vi "Offset_Loop.vi"(0 "Port":u16, 1 "LV_Variables":T1={"ACQPS"=25, "Config_Enable"=1, "Prescale"=1, "ADC"=enum."A", "Adc_Channel"=1, "Ref_Int/EXT"=FALSE}, 2 "ACQPS":u16[](array[numeric]), 5 "Core":u16, 7 "Pin_Config":i32, 11 "error in":errorcluster, 12 "Voltage":dbl[](array[numeric]), 14 "VREF_Measured":dbl=2.5 format="%#_13g") -> (4 "Port Number out":u16, 6 "Core Number out":u16, 8 "output array":string[][](array[string]), 13 "OFF+GAIN":string[][](array[string]), 15 "error out":errorcluster)   [LabVIEW 2019]
uses:
  Ctrls/ADC_LV_Variables.ctl
  Ctrls/ADC_CTRL.ctl
  <userlib>/_TI-LA/Reusable/CCS/APIs/Data/Polymorphics/Write Data To Symbol - U16.vi
  <userlib>/_TI-LA/Reusable/CCS/APIs/CCS.lvlib
  <vilib>/Analysis/NI_AALBase.lvlib
  common/Comman_nilesh/File_Write/Data_Logging.lvclass
  <userlib>/_TI-LA/Instr Drivers/Multimeter/Agilent 3446X Series/Agilent 3446X Series.lvlib
panel:
  out "AVG":dbl format="%0.2f"
  out "Array":dbl[](array[numeric])
  out "LV_Variables_out":T1={"ACQPS"=25, "Config_Enable"=1, "Prescale"=1, "ADC"=enum."A", "Adc_Channel"=1, "Ref_Int/EXT"=FALSE}
  in  "VISA_SGEN":refnum<visa-resource-name>="USB0::0x0957::0x1607::MY50001293::INSTR"
  out "standard deviation":dbl format="%0.2f"
  out "mean":dbl format="%0.2f"
  out "Waveform Graph":u16[](graph)
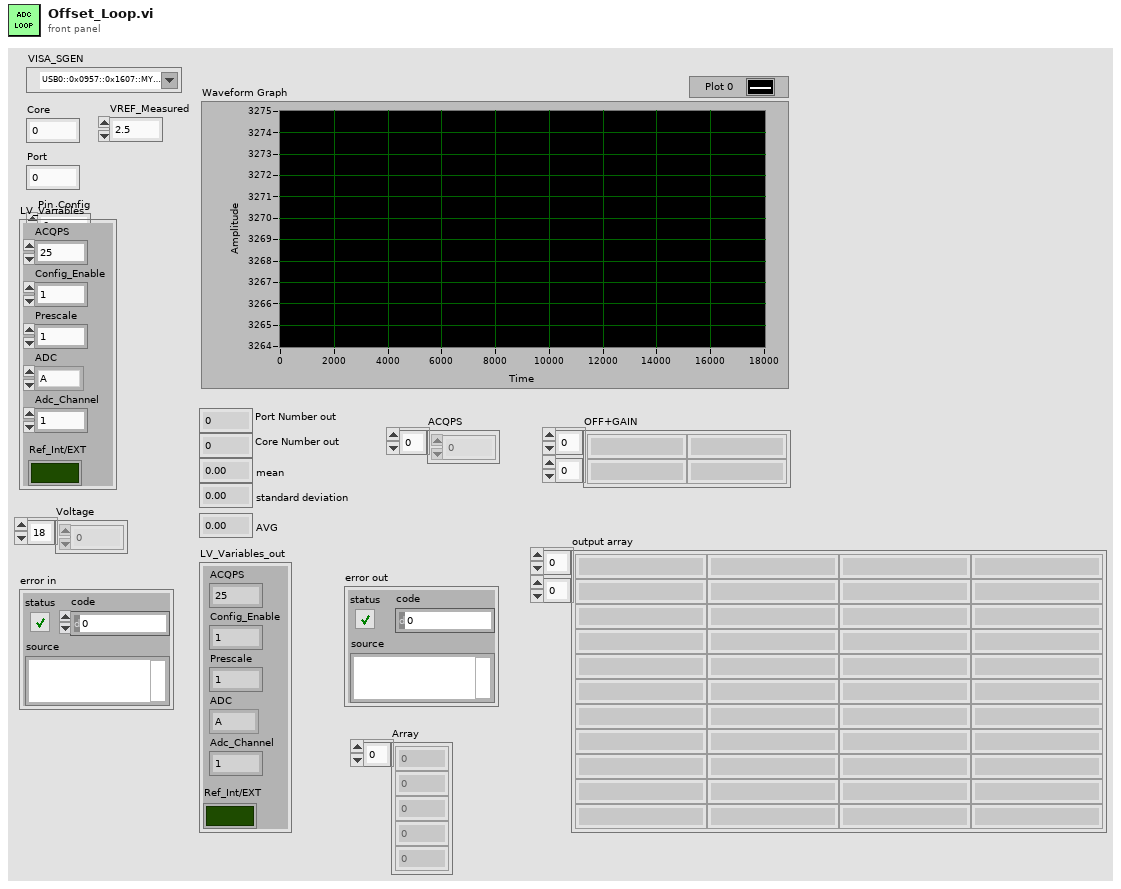
[diagram p1: front panel]
types:
  T1 = typedef "ADC_LV_Variables.ctl" = cluster{"ACQPS":u16, "Config_Enable":u16, "Prescale":u16, "ADC":T2, "Adc_Channel":u16, "Ref_Int/EXT":bool}
  T2 = typedef "ADC_CTRL.ctl" = enum16{"A", "B", "C"}
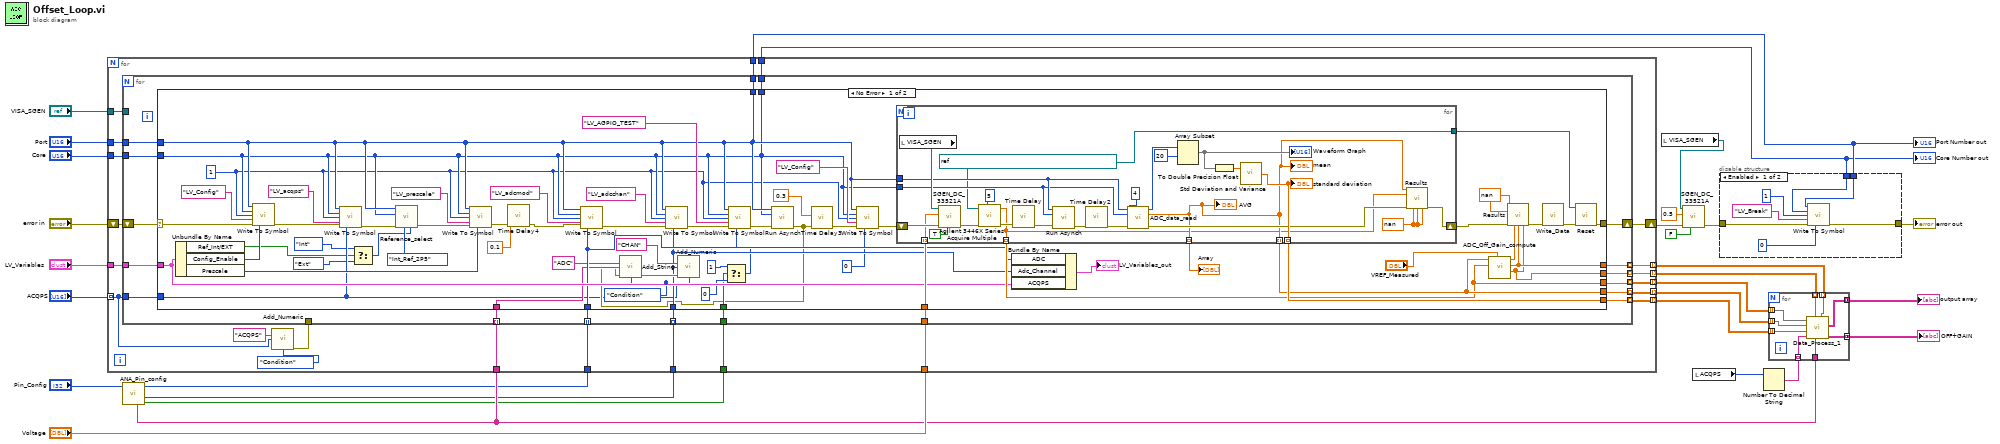
[diagram p0: block diagram]
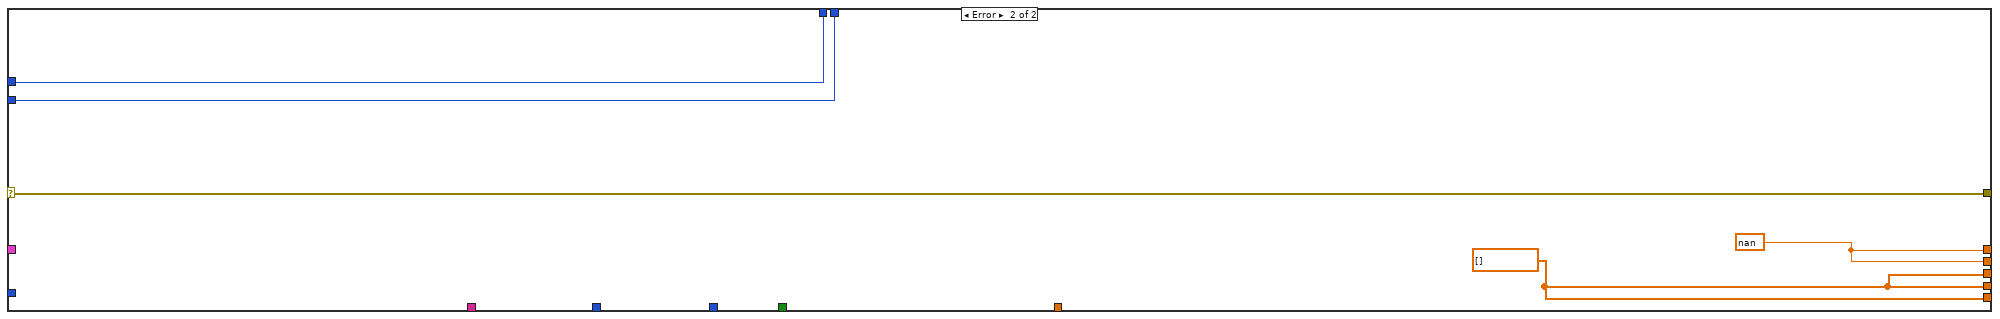
[diagram p3: hidden frame]
diagram:
  n1 = call "ANA_Pin_config.vi"("Pin_Config"="Pin_Config") -> ("Boolean"=w8:bool, "ADC_Channel"=w1:u16[], "ADC"=w2:T2[], "ADC+CH"=w9:string[])  [unwired: 7 in]
  n2 = for {
    tunnel: "Port" -> [w51]
    tunnel: "Core" -> [w50]
    tunnel: "LV_Variables" -> [w49]
    tunnel: [w47] -> w24
    tunnel: [w46] -> w23
    tunnel: w2 -> [w45]
    tunnel: w1 -> [w44]
    tunnel: "VISA_SGEN" -> [w43]
    tunnel: [w42] -> w10 mode=indexing
    tunnel: "Voltage" -> [w41]
    tunnel: [w40] -> w11 mode=indexing
    tunnel: [w39] -> w19 mode=indexing
    tunnel: [w38] -> w18 mode=indexing
    tunnel: [w37] -> w17 mode=indexing
    shift-right: [w48] -> w7
    shift-left: "error in" -> [w32]
    tunnel: "ACQPS" -> [w34] mode=indexing
    tunnel: w9 -> [w33]
    tunnel: w8 -> [w30]
    n3 = call "Add_Numeric.vi"("Name"="ACQPS", "Numeric_FC"=w34, "Type"=enum16{"Result", "Condition"}."Condition") -> ("error out"=w31:errorcluster)  [unwired: 11 in, 1 out]
    n4 = for {
      tunnel: w51 -> [w66]
      tunnel: w50 -> [w67]
      tunnel: w49 -> [w68]
      shift-right: [w69] -> w48
      shift-left: w32 -> [w63]
      tunnel: [w64] -> w46
      tunnel: [w65] -> w47
      tunnel: w45 -> [w55] mode=indexing
      tunnel: w44 -> [w62] mode=indexing
      tunnel: [w61] -> w38 mode=indexing
      tunnel: [w60] -> w37 mode=indexing
      tunnel: w41 -> [w59]
      tunnel: w43 -> [_]
      tunnel: [w58] -> w42 mode=indexing
      tunnel: [w57] -> w40 mode=indexing
      tunnel: [w56] -> w39 mode=indexing
      tunnel: w34 -> [w54]
      tunnel: w33 -> [w53] mode=indexing
      tunnel: w31 -> [_]
      tunnel: w30 -> [w52]
      n5 = case shown="No Error" w63 {
        selector: w63 -> [w123 w157]
        tunnel: [w98 w157] -> w69
        tunnel: w68 -> [w115 _]
        tunnel: w66 -> [w82 w159]
        tunnel: w67 -> [w81 w158]
        tunnel: [w82 w159] -> w65
        tunnel: [w81 w158] -> w64
        tunnel: w62 -> [w112 _]
        tunnel: [w121 w155] -> w61
        tunnel: [w122 w155] -> w60
        tunnel: w59 -> [w120 _]
        tunnel: [w92 w156] -> w58
        tunnel: [w91 w156] -> w57
        tunnel: [w119 w155] -> w56
        tunnel: w55 -> [w113 _]
        tunnel: w54 -> [w75 _]
        tunnel: w53 -> [w108 _]
        tunnel: w52 -> [w102 _]
        frame No Error {
          w94 = nan
          w111 = enum16{"Result", "Condition"}."Condition" ("Type")
          w80 = 1 ("Page")
          n6 = Unbundle By Name(w115) -> ("Ref_Int/EXT"=w73:bool, "Config_Enable"=w126:u16, "Prescale"=w118:u16)
          n7 = call-poly <userlib>:"Write To Symbol.vi"("Port Number"=w82, "Core Number"=w81, "Page"=w80, "Symbol Name"="LV_Config", "error in"=w123, "Write Data"=w126) -> ("error out"=w130:errorcluster)  [unwired: 7 in, 2 out]
          n8 = call-poly <userlib>:"Write To Symbol.vi"("Port Number"=w82, "Core Number"=w81, "Page"=w80, "Symbol Name"="LV_acqps", "error in"=w130, "Write Data"=w75) -> ("error out"=w101:errorcluster)  [unwired: 7 in, 2 out]
          n9 = Select(t=enum16{"Int", "Ext"}."Int" ("Ref_Sel(Int/Ext)"), s=w73, f=enum16{"Int", "Ext"}."Ext" ("Ref_Sel(Int/Ext)")) -> (s? t:f=w72:enum16{"Int", "Ext"})
          n10 = call "Reference_select.vi"("Ref_Sel(Int/Ext)"=w72, "INT_Ref_Sel"=enum16{"Int_Ref_1P65", "Int_Ref_2P5"}."Int_Ref_2P5", "error in"=w101, "Core Number"=w81, "Port Number"=w82) -> ("error out"=w100:errorcluster)  [unwired: 6 in]
          n11 = call-poly <userlib>:"Write To Symbol.vi"("Port Number"=w82, "Core Number"=w81, "Page"=w80, "Symbol Name"="LV_prescale", "error in"=w100, "Write Data"=w118) -> ("error out"=w79:errorcluster)  [unwired: 7 in, 2 out]
          n12 = call "Time Delay4"("error in (no error)"=w79, "Delay Time (s)"=0.1) -> ("error out"=w78:errorcluster)  [unwired: 9 in]
          n13 = call-poly <userlib>:"Write To Symbol.vi"("Port Number"=w82, "Core Number"=w81, "Page"=w80, "Symbol Name"="LV_adcmod", "error in"=w78, "Write Data"=w113) -> ("error out"=w109:errorcluster)  [unwired: 7 in, 2 out]
          n14 = call-poly <userlib>:"Write To Symbol.vi"("Port Number"=w82, "Core Number"=w81, "Page"=w80, "Symbol Name"="LV_adcchan", "error in"=w109, "Write Data"=w112) -> ("error out"=w107:errorcluster)  [unwired: 7 in, 2 out]
          n15 = Select(t=u16 1, s=w102, f=u16 0) -> (s? t:f=w105:u16)
          n16 = call-poly <userlib>:"Write To Symbol.vi"("Port Number"=w82, "Core Number"=w81, "Page"=w80, "Symbol Name"="LV_AGPIO_TEST", "error in"=w107, "Write Data"=w105) -> ("error out"=w88:errorcluster)  [unwired: 7 in, 2 out]
          n17 = call <userlib>:"Run Asynch.vi"("Port Number"=w82, "Core Number"=w81, "error in"=w88) -> ("error out"=w76:errorcluster)  [unwired: 10 in, 2 out]
          n18 = call "Add_String.vi"("Name"="ADC", "String_FC"=w108, "Error In"=w76, "Type"=w111) -> ("error out"=w116:errorcluster)  [unwired: 10 in, 1 out]
          n19 = call "Add_Numeric.vi"("Name"="CHAN", "Numeric_FC"=w112, "Error In"=w116, "Type"=w111) -> ()  [unwired: 10 in, 2 out]
          n20 = call "Time Delay3"("error in (no error)"=w76, "Delay Time (s)"=0.3) -> ("error out"=w86:errorcluster)  [unwired: 9 in]
          n21 = call-poly <userlib>:"Write To Symbol.vi"("Port Number"=w82, "Core Number"=w81, "Page"=w80, "Symbol Name"="LV_Config", "error in"=w86, "Write Data"=u16 0) -> ("error out"=w85:errorcluster)  [unwired: 7 in, 2 out]
          n22 = for {
            tunnel: w82 -> [w143]
            tunnel: w81 -> [w142]
            tunnel: [w132] -> w121 mode=indexing
            tunnel: [w149] -> w122 mode=indexing
            shift-right: [w135] -> w96
            shift-left: w85 -> [w146]
            tunnel: w120 -> [w141] mode=indexing
            tunnel: [w131] -> w119 mode=indexing
            tunnel: [w137] -> w97
            tunnel: [w132] -> w90 mode=indexing
            w134 = nan
            w137 = refnum<visa-resource-name> "USB0::0x2A8D::0x1301::MY57222838::INSTR" ("VISA resource name")
            n23 = local read "VISA_SGEN"() -> (w148:refnum<visa-resource-name>)
            n24 = call "SGEN_DC_33521A.vi"("Enable Output (T: Enable)"=TRUE, "error in (no error)"=w146, "DC Offset (0 V)"=w141, "VISA_SGEN"=w148) -> ("error out"=w140:errorcluster)  [unwired: 7 in]
            n25 = call "Agilent 3446X Series Acquire Multiple.vi"("Sample Count (1)"=5, "error in (no error)"=w140, "VISA resource name"=w137) -> ("error out"=w139:errorcluster, "mean"=w131:dbl)  [unwired: 6 in, 1 out]
            n26 = call "Time Delay"("error in (no error)"=w139) -> ("error out"=w147:errorcluster)  [unwired: 10 in]
            n27 = call <userlib>:"Run Asynch.vi"("Port Number"=w143, "Core Number"=w142, "error in"=w147) -> ("error out"=w145:errorcluster)  [unwired: 10 in, 2 out]
            n28 = call "Time Delay2"("error in (no error)"=w145) -> ("error out"=w144:errorcluster)  [unwired: 10 in]
            n29 = call "ADC_data_read.vi"("Port Number"=w143, "Core Number"=w142, "Page"=4 ("No_Iterations"), "error in (no error)"=w144) -> ("Read Data[]"=w151:u16[], "Read Data"=w132:dbl, "error out"=w136:errorcluster)  [unwired: 9 in]
            "mean" <- w132
            "AVG" <- w132
            n30 = Array Subset(array=w151, index=20) -> (w150:u16[])  [unwired: 1 in]
            "Waveform Graph" <- w150
            n31 = To Double Precision Float(number=w150) -> (double precision float=w153:dbl[])
            n32 = call <vilib>:"Std Deviation and Variance.vi"("X"=w153) -> ("standard deviation"=w149:dbl)  [unwired: 1 in, 2 out]
            "standard deviation" <- w149
            n33 = call "Results.vi"("Code"=w132, "Voltage"=w131, "Error In"=w136, "Slope"=w134, "Offset_Error"=w134, "Gain_error"=w134) -> ("error out"=w135:errorcluster)  [unwired: 9 in]
          }
          "Array" <- w90
          n34 = Bundle By Name(cluster=w115, "ADC"=w113, "Adc_Channel"=w112, "ACQPS"=w75) -> (→"LV_Variables_out":T1)
          n35 = call "ADC_Off_Gain_compute.vi"("VREF_Measured"="VREF_Measured", "Voltage_Array"=w119, "Code"=w121) -> ("Gain_Error_(LSB)"=w91:dbl, "Offset_Error"=w92:dbl, "slope"=w93:dbl)  [unwired: 5 in, 1 out]
          n36 = call "Results.vi"("Code"=w94, "Voltage"=w94, "Error In"=w96, "Slope"=w93, "Offset_Error"=w92, "Gain_error"=w91) -> ("error out"=w95:errorcluster)  [unwired: 9 in]
          n37 = call "Write_Data.vi"("Error In"=w95) -> ("error out"=w99:errorcluster)  [unwired: 9 in, 1 out]
          n38 = call <userlib>:"Reset.vi"("error in (no error)"=w99, "VISA resource name"=w97) -> ("error out"=w98:errorcluster)  [unwired: 8 in, 1 out]
        }
        frame Error {
          w156 = nan
          w155 = dbl[] []
        }
      }
    }
  }
  "Core Number out" <- w23
  "Port Number out" <- w24
  n39 = local read "VISA_SGEN"() -> (w5:refnum<visa-resource-name>)
  n40 = call "SGEN_DC_33521A.vi"("Enable Output (T: Enable)"=FALSE, "error in (no error)"=w7, "DC Offset (0 V)"=0.5, "VISA_SGEN"=w5) -> ("error out"=w6:errorcluster)  [unwired: 7 in]
  n41 = local read "ACQPS"() -> (w14:u16[])
  n42 = disable-structure shown="Enabled" {
    disable-tunnel: w6 -> [w163 w167]
    disable-tunnel: [w160 w167] -> w25
    disable-tunnel: w24 -> [w162 _]
    disable-tunnel: w23 -> [w161 _]
    frame Enabled {
      n43 = call-poly <userlib>:"Write To Symbol.vi"("Port Number"=w162, "Core Number"=w161, "Page"=1, "Symbol Name"="LV_Break", "error in"=w163, "Write Data"=u16 0) -> ("error out"=w160:errorcluster)  [unwired: 7 in, 2 out]
    }
    frame Disabled {
    }
  }
  "error out" <- w25
  n44 = Number To Decimal String(number=w14) -> (decimal integer string=w13:string[])  [unwired: 1 in]
  n45 = for {
    tunnel: w19 -> [w176] mode=indexing
    tunnel: w18 -> [w175] mode=indexing
    tunnel: w17 -> [w174] mode=indexing
    tunnel: w9 -> [w173]
    tunnel: w13 -> [w172] mode=indexing
    tunnel: [w171] -> w15 mode=concatenating
    tunnel: [w170] -> w12 mode=concatenating
    tunnel: w11 -> [w169] mode=indexing
    tunnel: w10 -> [w168] mode=indexing
    n46 = call "Data_Process_1.vi"("Offset_Error"=w168, "ADC+CH"=w173, "Gain_Error"=w169, "ACQPS"=w172, "Std_Deviation"=w174, "Mean"=w175, "Vin_Measured"=w176) -> ("OFF+GAIN"=w170:string[][], "output array"=w171:string[][])  [unwired: 3 in]
  }
  "output array" <- w15
  "OFF+GAIN" <- w12
